vi "previousOff.vi"(1 "add prev":bool, 2 "in":dbl[](array[numeric])) -> (0 "out":dbl[](array[numeric]))   [LabVIEW 2009]
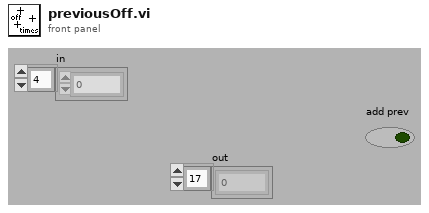
[diagram p1: front panel]
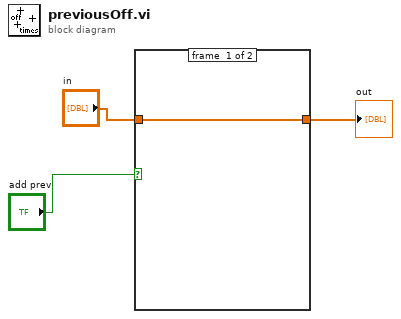
[diagram p0: block diagram]
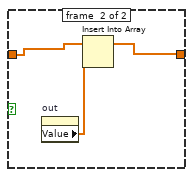
[diagram p2: hidden frame]
diagram:
  n1 = case shown="True" "add prev" {
    tunnel: "in" -> [w4 w7]
    tunnel: [w4 w6] -> w1
    frame #0 {
    }
    frame #1 {
      n2 = property on="out" class="Arr (strikt)"() -> ("Value"=w5:dbl[])  [unwired: 2 in, 2 out]
      n3 = Insert Into Array(array=w7, new element=w5) -> (w6:dbl[])  [unwired: 1 in]
    }
  }
  "out" <- w1
